vi "Binary String to HEX.vi"(10 "Bin Length":i32=16, 11 "Bin String in":string) -> (3 "hex integer string":string)   [LabVIEW 2016]
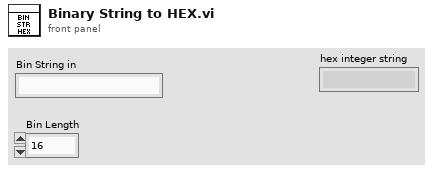
[diagram p1: front panel]
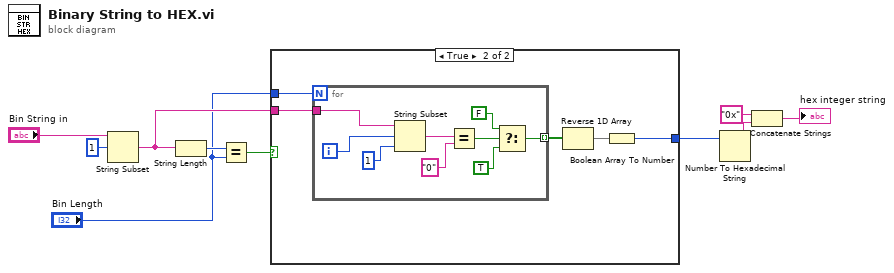
[diagram p0: block diagram]
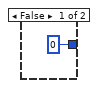
[diagram p2: hidden frame]
diagram:
  n1 = String Subset(string="Bin String in", offset (0)=1) -> (substring=w6:string)  [unwired: 1 in]
  n2 = String Length(string=w6) -> (length=w8:i32)
  n3 = Equal?(x=w8, y="Bin Length") -> (x = y?=w7:bool)
  n4 = case shown="True" w7 {
    tunnel: w6 -> [_ w15]
    tunnel: "Bin Length" -> [_ w16]
    tunnel: [u32 0 w12] -> w4
    frame False {
    }
    frame True {
      n5 = for {
        N: w16 -> [_]
        tunnel: w15 -> [w25]
        tunnel: [w17] -> w14 mode=indexing
        i -> [w23]
        n6 = String Subset(string=w25, offset (0)=w23, length (rest)=1 ("length (rest)")) -> (substring=w22:string)
        n7 = Equal?(x=w22, y="0") -> (x = y?=w20:bool)
        n8 = Select(t=FALSE, s=w20, f=TRUE) -> (s? t:f=w17:bool)
      }
      n9 = Reverse 1D Array(array=w14) -> (reversed array=w13:bool[])
      n10 = Boolean Array To Number(Boolean array=w13) -> (number=w12:u32)
    }
  }
  n11 = Number To Hexadecimal String(2:w4) -> (0:w3:string)  [unwired: 1 in]
  n12 = Concatenate Strings("0x" ("string"), w3) -> (→"hex integer string":string)
